vi "Wait.vi"(9 "PS VISA in":refnum<visa-resource-name>, 11 "PS error in":errorcluster caption="PS error in (no error)", 12 "Wait Filepath":path=path "C:/Users/ga11/Desktop/VI/results/3PtestChrgRest.lvm" caption="Filename", 13 "Wait time":dbl) -> (10 "PS Visa Out":refnum<visa-resource-name>, 15 "PS error out":errorcluster)   [LabVIEW 2020]
uses:
  Drivers-IT-M3400/IT-M3400.lvlib
panel:
  out "Read Current(A)":dbl format="%.2g"
  out "Read Voltage(V)":dbl format="%.2g"
  out "loop":dbl
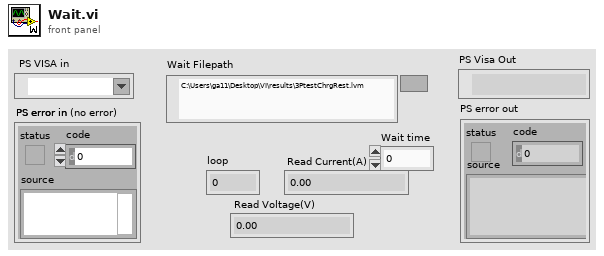
[diagram p1: front panel]
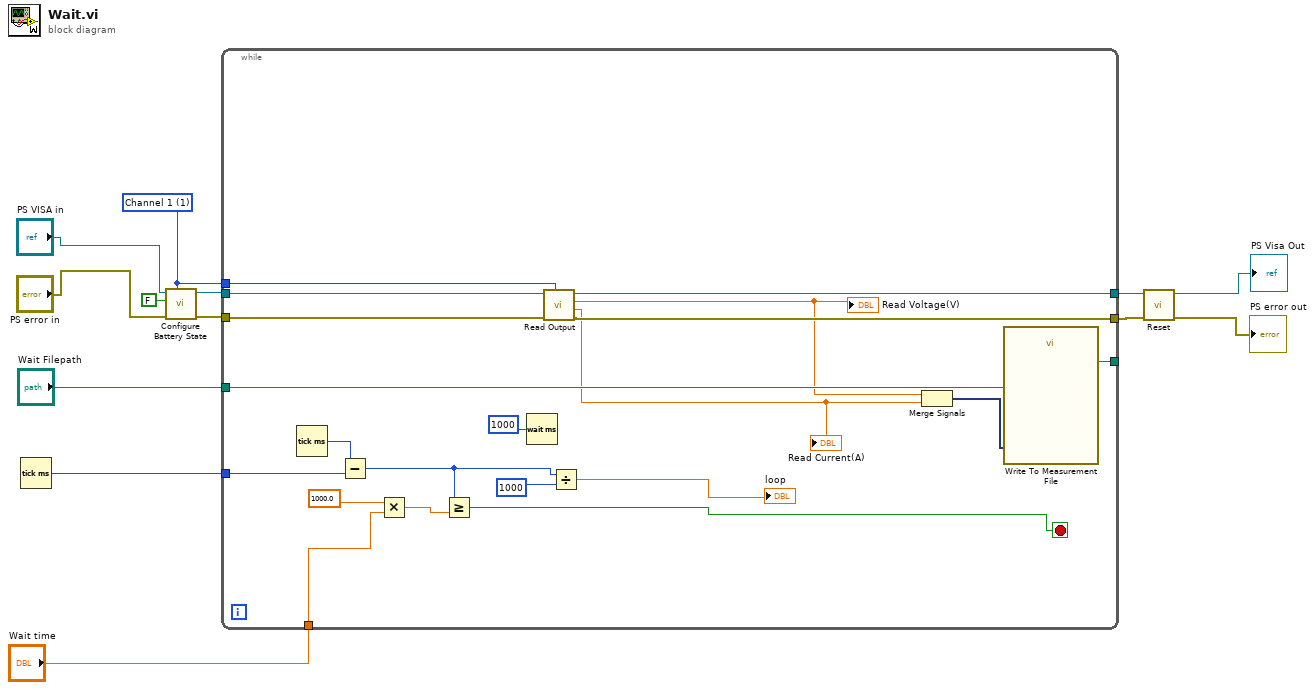
[diagram p0: block diagram]
diagram:
  w3 = 1 items=["Channel 1"=1, "Channel 2"=2, "Channel 3"=3, "Channel 4"=4, "Channel 5"=5, "Channel 6"=6, "Channel 7"=7, "Channel 8"=8, "Channel 8"=9, "Channel 10"=10, "Channel 11"=11, "Channel 12"=12, "Channel 13"=13, "Channel 14"=14, "Channel 15"=15, "Channel 16"=16] ("Channel")
  n1 = Tick Count (ms)() -> (millisecond timer value=w12:u32)
  n2 = call "Configure Battery State.vi"("Channel"=w3, "error in"="PS error in", "State"=FALSE, "VISA resource name"="PS VISA in") -> ("error out"=w5:errorcluster, "VISA resource name out"=w6:refnum<visa-resource-name>)  [unwired: 6 in]
  n3 = while {
    tunnel: "Wait time" -> [w30]
    tunnel: [w27] -> _
    tunnel: w12 -> [w26]
    tunnel: "Wait Filepath" -> [w25]
    tunnel: [w21] -> w2
    tunnel: [w20] -> w1
    tunnel: w6 -> [w18]
    tunnel: w5 -> [w17]
    tunnel: w3 -> [w16]
    stop <- w31 stop-if-true
    n4 = Tick Count (ms)() -> (millisecond timer value=w32:u32)
    n5 = Subtract(x=w32, y=w26) -> (x-y=w24:u32)
    n6 = Multiply(x=1000.0, y=w30) -> (x*y=w28:dbl)
    n7 = Greater Or Equal?(x=w24, y=w28) -> (x >= y?=w31:bool)
    n8 = Wait (ms)(milliseconds to wait=1000) -> ()  [unwired: 1 out]
    n9 = call "Read Output.vi"("Channel"=w16, "error in"=w17, "VISA resource name"=w18) -> ("error out"=w20:errorcluster, "Read Current(A)"=w15:dbl, "Read Voltage(V)"=w14:dbl, "VISA resource name out"=w21:refnum<visa-resource-name>)  [unwired: 5 in]
    "Read Voltage(V)" <- w14
    "Read Current(A)" <- w15
    n10 = Divide(x=w24, y=1000) -> (x/y=→"loop":dbl)
    n11 = Merge Signals "Merge Signals"(w14, w15) -> (w22:dynamicdata)
    n12 = call "Write To Measurement File"("Signals"=w22, "Filename"=w25) -> ("Filename Out"=w27:path)  [unwired: 15 in, 2 out]
  }
  n13 = call "Reset.vi"("error in"=w1, "VISA resource name"=w2) -> ("error out"=→"PS error out":errorcluster, "VISA resource name out"=→"PS Visa Out":refnum<visa-resource-name>)  [unwired: 8 in]
